vi "test 4- NonCSMCallsChainMode_UseAPI.vi"(8 "error in (no error)":errorcluster, 11 "TestCase in":refnum<class "testcase-SyncMessage.lvclass">) -> (0 "error out":errorcluster, 3 "TestCase out":refnum<class "testcase-SyncMessage.lvclass">)   [LabVIEW 2017, in "testcase-SyncMessage.lvclass"]
uses:
  testcase-SyncMessage.lvclass
  src/user.lib/_NEVSTOP/Communicable State Machine(CSM)/_Support/Typedef/_CSM_MODE.ctl
  _support/SyncMessage_CSM_Callee_ForChainMode.vi
  <vilib>/addons/_JKI Toolkits/VI Tester/TestCase.llb/TestCase.lvclass
  src/user.lib/_NEVSTOP/Communicable State Machine(CSM)/Communicable State Machine.lvlib
  C:/Program Files (x86)/National Instruments/LabVIEW 2017/vi.lib/addons/_JKI Toolkits/VI Tester/TestCase.llb/TestCase.lvclass
panel:
  out "Array 2":T2(array[cluster])
  in  "All?":bool
  out "Array":string[](array[string])
  out ">> Msg/Rep's CSM >>":string
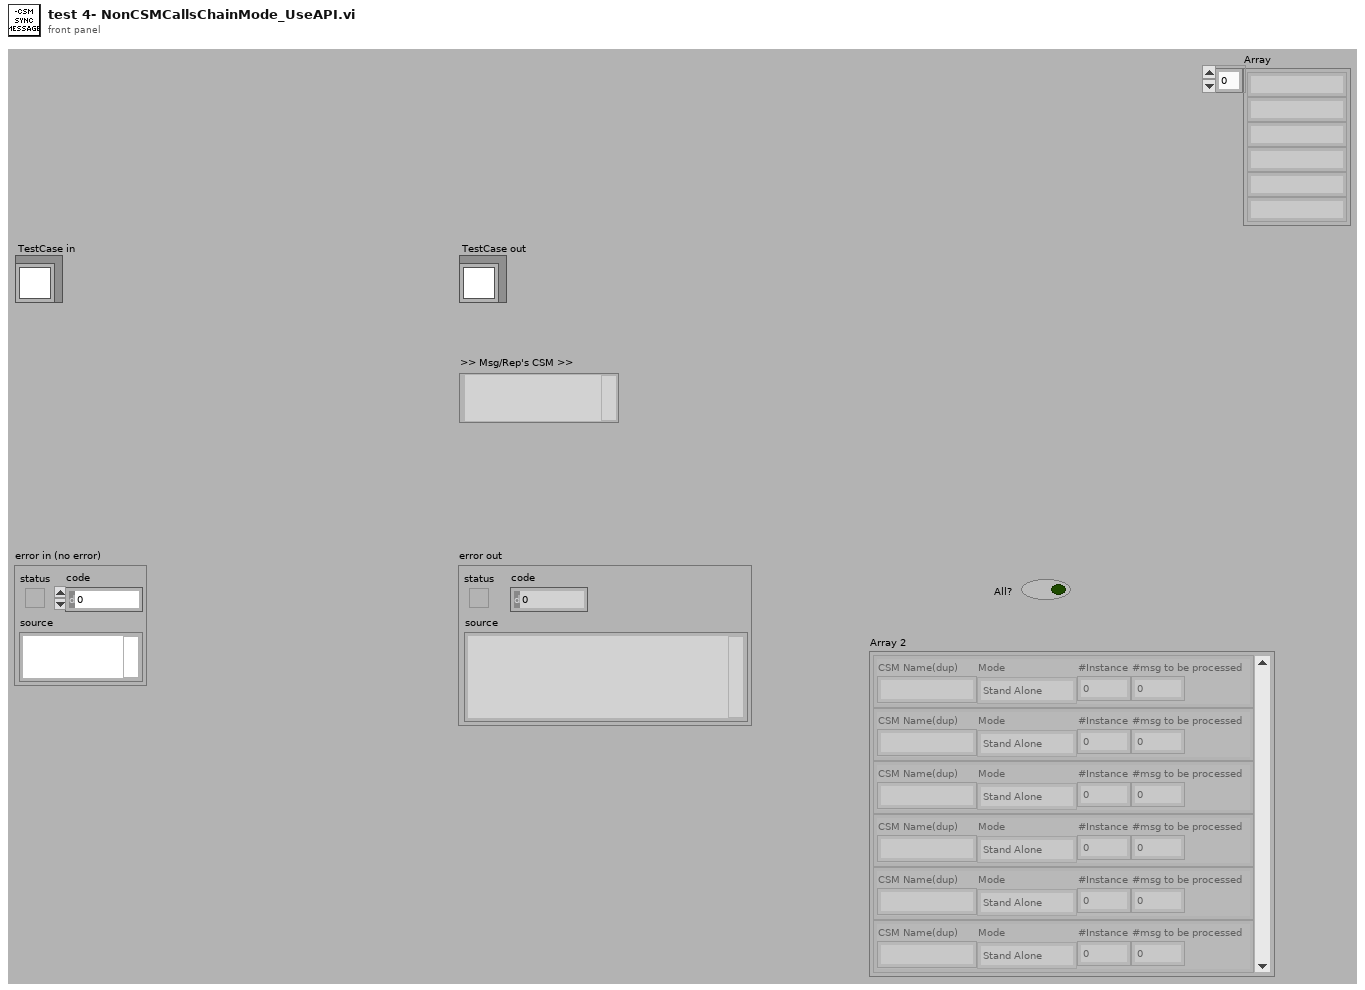
[diagram p1: front panel]
types:
  T1 = typedef "Communicable State Machine.lvlib/_CSM_MODE.ctl" = enum16{"Not Exist", "Stand Alone", "CSM", "Worker", "Worker Agent", "Chain Node", "Chain"}
  T2 = cluster{"CSM Name(dup)":string, "Mode":T1, "#Instance":i32, "#msg to be processed":i32}[]
  T3 = cluster{"CSM Name (Dup)":string, "Mode":T1, "#Instance":i32, "#Elements In Queue":i32}
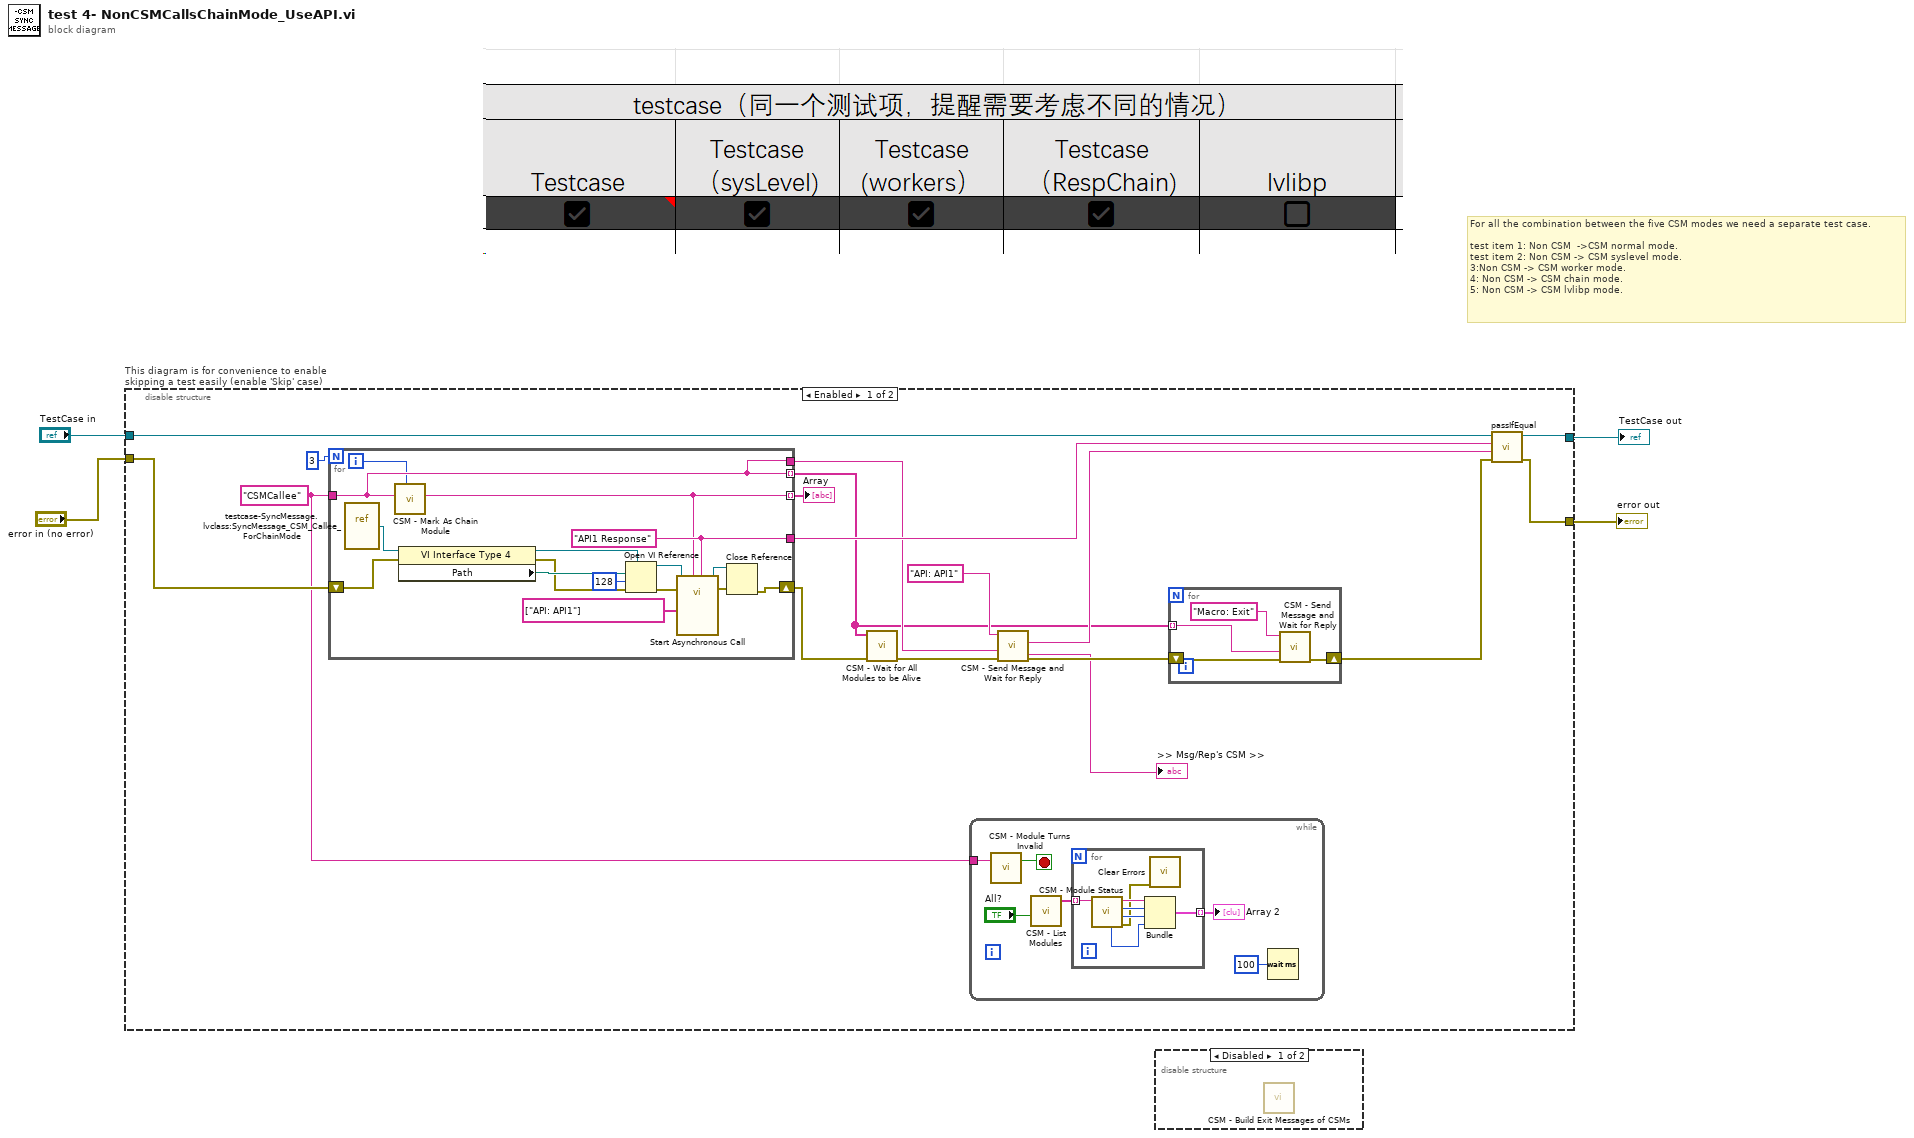
[diagram p0: block diagram]
diagram:
  # "For all the combination between the five CSM modes we need a separate test case.\n\ntest item 1: Non CSM  ->CSM normal mode.\ntest item 2: Non CSM -> CSM syslevel mode.\n3:Non CSM -> CSM worker mode.\n4: Non CSM -> CSM chain mode.\n5: Non CSM -> CSM lvlibp mode."
  n1 = disable-structure "This diagram is for convenience to enable skipping a test easily (enable 'Skip' case)" shown="Enabled" {
    disable-tunnel: "TestCase in" -> [w21 w58]
    disable-tunnel: [w20 w56] -> w2
    disable-tunnel: [w19 w57] -> w1
    disable-tunnel: "error in (no error)" -> [w14 w55]
    frame Enabled {
      w5 = "CSMCallee"
      n2 = for {
        N: 3 -> [_]
        tunnel: [w40] -> w13
        shift-right: [w39] -> w11
        shift-left: w14 -> [w41]
        tunnel: w5 -> [w37]
        tunnel: [w37] -> w8 mode=indexing
        tunnel: [w37] -> w9
        tunnel: [w36] -> w6 mode=indexing
        i -> [w35]
        w40 = "API1 Response" ("API response in")
        n3 = vi-ref "testcase-SyncMessage.lvclass:SyncMessage_CSM_Callee_ForChainMode.vi"() -> (w49:refnum<vi>)
        n4 = call "CSM - Mark As Chain Module.vi"("Order"=w35, "CSM Name"=w37) -> ("CSM Name (Marked As Chain)"=w36:string)  [unwired: 8 in]
        n5 = property class="VI Interface Type 4"(reference=w49, error in=w41) -> (reference out=w45:refnum<vi>, error out=w47:errorcluster, "Path"=w48:path)
        n6 = Open VI Reference(type specifier VI Refnum (for type only)=w45, vi path=w48, options=128, error in (no error)=w47) -> (vi reference=w46:refnum<vi>, error out=w50:errorcluster)  [unwired: 2 in]
        n7 = call-by-ref "Start Asynchronous Call"(reference=w46, error in=w50, "API response in"=w40, "Name (\"\" to Use UUID)"=w36, "Allowed Messages (Empty for All)"=string[] ["API: API1"]) -> (reference out=w43:refnum<vi>, error out=w44:errorcluster)  [unwired: 9 in]
        n8 = Close Reference(reference=w43, error in (no error)=w44) -> (error out=w39:errorcluster)
      }
      "Array" <- w6
      n9 = call "CSM - Wait for All Modules to be Alive.vi"("Error In"=w11, "CSM Names"=w8) -> ("error out"=w7:errorcluster)  [unwired: 7 in, 2 out]
      n10 = while {
        tunnel: w5 -> [w24]
        stop <- w25 stop-if-true
        n11 = call "CSM - Module Turns Invalid.vi"("CSM Name"=w24) -> ("Turn Invalid (Exit)?"=w25:bool)  [unwired: 2 in]
        n12 = call "CSM - List Modules.vi"("With Instance? (F)"="All?") -> ("Module Names"=w26:string[])  [unwired: 9 in, 1 out]
        n13 = for {
          tunnel: w26 -> [w34] mode=indexing
          tunnel: [w29] -> w27 mode=indexing
          n14 = call "CSM - Module Status.vi"("CSM Name"=w34) -> ("error out"=w28:errorcluster, "#Instance"=w31:i32, "Mode"=w32:T1, "CSM Name (Dup)"=w33:string, "#Elements In Queue"=w30:i32)  [unwired: 6 in]
          n15 = Bundle("CSM Name (Dup)"=w33, "Mode"=w32, "#Instance"=w31, "#Elements In Queue"=w30) -> (w29:T3)  [unwired: 1 in]
          n16 = call <vilib>:"Clear Errors.vi"("error in (no error)"=w28) -> ()  [unwired: 5 in, 2 out]
        }
        "Array 2" <- w27
        n17 = Wait (ms)(milliseconds to wait=u32 100) -> ()  [unwired: 1 out]
      }
      n18 = call "CSM - Send Message and Wait for Reply.vi"("Error In (No Error)"=w7, "Target Module"=w9, "State"="API: API1") -> ("error out"=w15:errorcluster, "Response"=w16:string, ">> Msg/Rep's CSM >>"=→">> Msg/Rep's CSM >>":string)  [unwired: 6 in]
      n19 = for {
        shift-right: [w53] -> w18
        shift-left: w15 -> [w54]
        tunnel: w8 -> [w51] mode=indexing
        n20 = call "CSM - Send Message and Wait for Reply.vi"("Error In (No Error)"=w54, "Target Module"=w51, "State"="Macro: Exit") -> ("error out"=w53:errorcluster)  [unwired: 6 in, 2 out]
      }
      n21 = call-dynamic "passIfEqual.vi"("error in (no error)"=w18, "y"=w16, "x"=w13, "TestCase in"=w21) -> ("error out"=w19:errorcluster, "TestCase out"=w20:refnum<class "testcase-SyncMessage.lvclass">)  [unwired: 6 in]
    }
    frame Disabled {
      # "skip test result while test is under development"
      n22 = call <vilib>:"skip.vi"("error in (no error)"=w55, "TestCase in"=w58) -> ("error out"=w57:errorcluster, "TestCase out"=w56:refnum<class "testcase-SyncMessage.lvclass">)  [unwired: 8 in]
    }
  }
  "error out" <- w1
  "TestCase out" <- w2
  n23 = disable-structure shown="Disabled" {
    frame Disabled {
      n24 = call "CSM - Build Exit Messages of CSMs.vi"() -> ()  [unwired: 15 in, 1 out]
    }
    frame Enabled {
    }
  }
